vi "KB-Laser 寻找內圆.vi"(6 "offset Y":sgl, 7 "旧ROI":T1 {"Contours"."Type" items=["No Selection", "Point", "Line", "Rectangle", "Oval", "Polygon", "Freehand Region", "Annulus", "Unused2", "Unused3", "Broken Line", "Freehand Line", "Rotated Rectangle"]}, 8 "內环半径":i32=17, 10 "旧圆心":T2 {"Average SNR (dB)" format="%.2f"; "Average Strength" format="%.2f"; "Roundness (Real-World)" format="%.2f"; "Radius (Real-World)" format="%.2f"; "Center (Real-World)"."Y" format="%.2f"; "Center (Real-World)"."X" format="%.2f"; "Radius (Pixels)" format="%.2f"; "Center (Pixels)"."Y" format="%.2f"; "Center (Pixels)"."X" format="%.2f"}, 11 "新圆心":T2 {"Average SNR (dB)" format="%.2f"; "Average Strength" format="%.2f"; "Roundness (Real-World)" format="%.2f"; "Radius (Real-World)" format="%.2f"; "Center (Real-World)"."Y" format="%.2f"; "Center (Real-World)"."X" format="%.2f"; "Radius (Pixels)" format="%.2f"; "Center (Pixels)"."Y" format="%.2f"; "Center (Pixels)"."X" format="%.2f"}) -> (0 "范围内？":bool, 1 "Radius (Pixels)":dbl, 2 "Center (Pixels)":cluster{"X":sgl, "Y":sgl}, 3 "ROI Descriptor":T1 {"Contours"."Type" items=["No Selection", "Point", "Line", "Rectangle", "Oval", "Polygon", "Freehand Region", "Annulus", "Unused2", "Unused3", "Broken Line", "Freehand Line", "Rotated Rectangle"]})   [LabVIEW 2015]
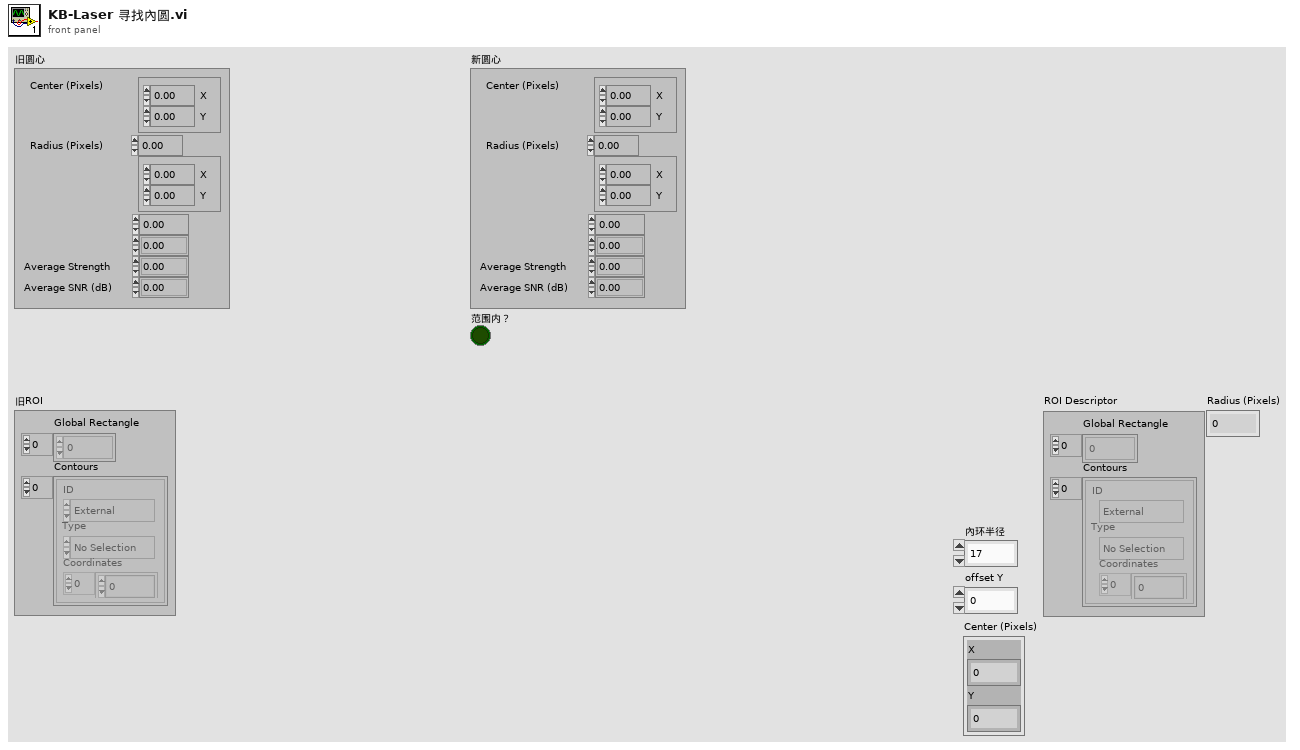
[diagram p1: front panel]
types:
  T1 = typedef "ROI Descriptor" = cluster{"Global Rectangle":i32[], "Contours":cluster{"ID":enum32{"External", "Internal"}, "Type":u32, "Coordinates":i32[]}[]}
  T2 = cluster{"Center (Pixels)":cluster{"X":sgl, "Y":sgl}, "Radius (Pixels)":dbl, "Center (Real-World)":cluster{"X":sgl, "Y":sgl}, "Radius (Real-World)":dbl, "Roundness (Real-World)":dbl, "Average Strength":dbl, "Average SNR (dB)":dbl}
  T3 = typedef "IMAQ Circle" = cluster{"Center X":i32, "Center Y":i32, "Inner Radius":i32, "Outer Radius":i32, "Start Angle":dbl, "End Angle":dbl}
  T4 = cluster{"ID":enum32{"External", "Internal"}, "Type":u32, "Coordinates":i32[]}[]
  T5 = cluster{"ID":enum32{"External", "Internal"}, "Type":u32, "Coordinates":i32[]}
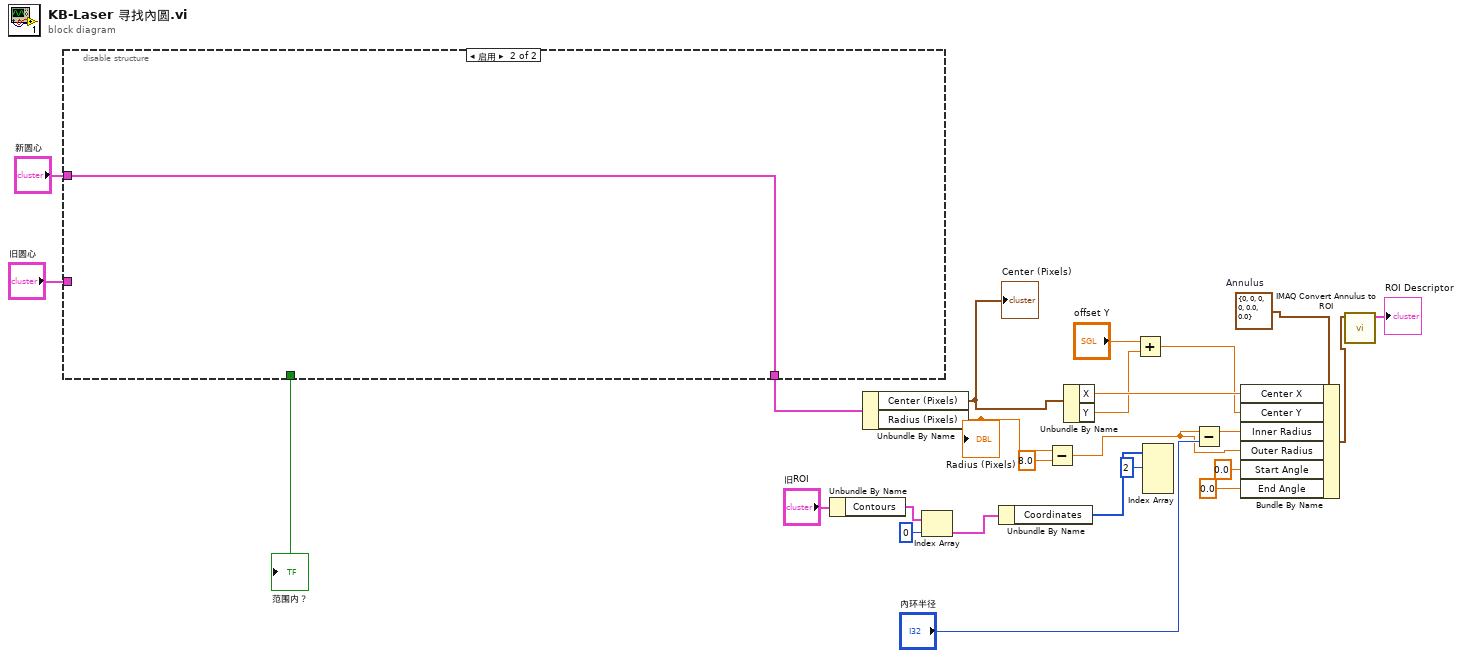
[diagram p0: block diagram]
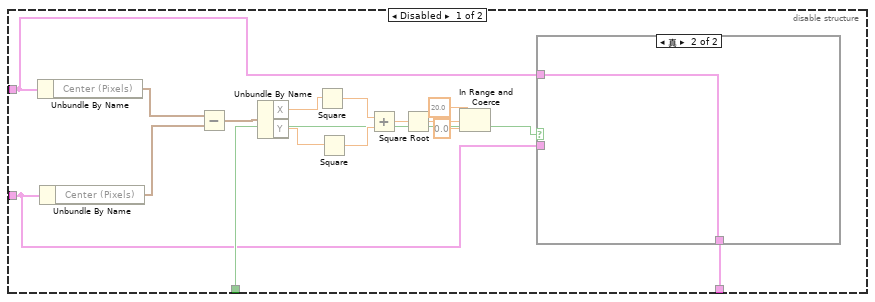
[diagram p2: hidden frame]
diagram:
  w22 = T3 {"Center X"=0, "Center Y"=0, "Inner Radius"=0, "Outer Radius"=0, "Start Angle"=0.0, "End Angle"=0.0}  # Annulus
  n1 = disable-structure shown="启用" {
    disable-tunnel: [w29 _] -> w25
    disable-tunnel: "新圆心" -> [w28 w43]
    disable-tunnel: "旧圆心" -> [w27 _]
    disable-tunnel: [w26 w43] -> w8
    frame Disabled {
      n2 = Unbundle By Name(w28) -> ("Center (Pixels)"=w40:cluster{"X":sgl, "Y":sgl})
      n3 = Unbundle By Name(w27) -> ("Center (Pixels)"=w39:cluster{"X":sgl, "Y":sgl})
      n4 = Subtract(x=w40, y=w39) -> (x-y=w38:cluster{"X":sgl, "Y":sgl})
      n5 = Unbundle By Name(w38) -> ("X"=w37:sgl, "Y"=w36:sgl)
      n6 = Square(x=w37) -> (x^2=w35:sgl)
      n7 = Square(x=w36) -> (x^2=w34:sgl)
      n8 = Add(x=w35, y=w34) -> (x+y=w33:sgl)
      n9 = Square Root(x=w33) -> (sqrt(x)=w32:sgl)
      n10 = In Range and Coerce(upper limit=sgl 20.0 ("上限"), x=w32, lower limit=sgl 0.0 ("下限")) -> (In Range?=w29:bool)  [unwired: 1 out]
      n11 = case shown="真" w29 {
        tunnel: w28 -> [w41 w42]
        tunnel: w27 -> [_ _]
        tunnel: [w41 w42] -> w26
        frame False {
        }
        frame True {
        }
      }
    }
    frame Enabled {
    }
  }
  "范围内？" <- w25
  n12 = Unbundle By Name("旧ROI") -> ("Contours"=w20:T4)
  n13 = Unbundle By Name(w8) -> ("Center (Pixels)"=w9:cluster{"X":sgl, "Y":sgl}, "Radius (Pixels)"=w4:dbl)
  "Center (Pixels)" <- w9
  "Radius (Pixels)" <- w4
  n14 = Index Array(array=w20, index=0 ("索引")) -> (element=w18:T5)
  n15 = Unbundle By Name(w18) -> ("Coordinates"=w17:i32[])
  n16 = Subtract(x=w4, y=8.0) -> (x-y=w3:dbl)
  n17 = Unbundle By Name(w9) -> ("X"=w21:sgl, "Y"=w12:sgl)
  n18 = Add(x="offset Y", y=w12) -> (x+y=w10:sgl)
  n19 = Index Array(array=w17, index #1=2 ("索引")) -> ()  [unwired: 3 in, 4 out]
  n20 = Subtract(x=w3, y="內环半径") -> (x-y=w13:dbl)
  n21 = Bundle By Name(cluster=w22, "Center X"=w21, "Center Y"=w10, "Inner Radius"=w13, "Outer Radius"=w3, "Start Angle"=0.0, "End Angle"=0.0) -> (w15:T3)
  n22 = call "IMAQ Convert Annulus to ROI"("Annulus"=w15) -> ("ROI Descriptor"=→"ROI Descriptor":T1)  [unwired: 8 in, 1 out]
